vi "ProjectInstance.vi"() -> ()   [LabVIEW 2016, in "test_Setup.lvlib"]
uses:
  test_Setup.lvlib
  <vilib>/addons/_JKI Toolkits/Caraya/classes/Assert/Assert Equal Value_Variant.vi
  <vilib>/addons/_JKI Toolkits/Caraya/classes/Test/Test.lvclass
  <vilib>/addons/_JKI Toolkits/Caraya/classes/Assert/Assert.lvclass
panel:
  out "error out":errorcluster
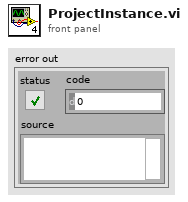
[diagram p1: front panel]
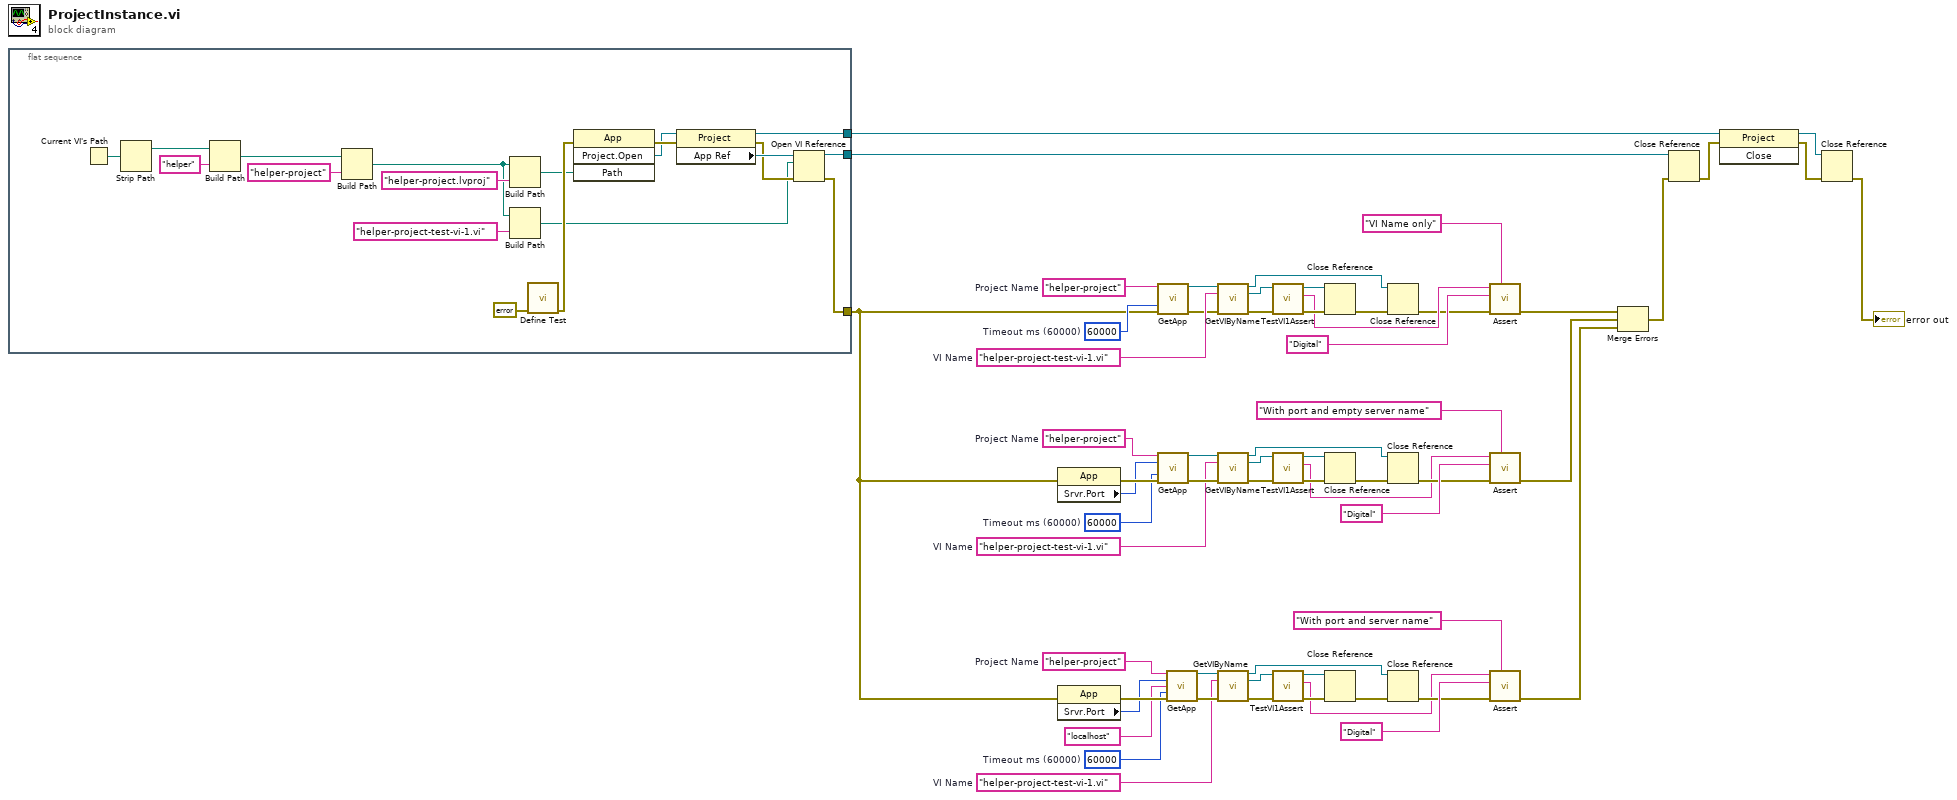
[diagram p0: block diagram]
diagram:
  w1 = "helper-project"  # Project Name
  w2 = "helper-project"  # Project Name
  w3 = "helper-project"  # Project Name
  w7 = 60000  # Timeout ms (60000)
  w10 = "helper-project-test-vi-1.vi"  # VI Name
  w22 = 60000  # Timeout ms (60000)
  w21 = "helper-project-test-vi-1.vi"  # VI Name
  w43 = 60000  # Timeout ms (60000)
  w41 = "helper-project-test-vi-1.vi"  # VI Name
  n1 = flat-sequence {
    tunnel: [w79] -> w5
    tunnel: [w78] -> w61
    tunnel: [w66] -> w60
    frame #0 {
      n2 = Current VI's Path() -> (path=w77:path)
      n3 = Strip Path(path=w77) -> (stripped path=w76:path)  [unwired: 1 out]
      n4 = Build Path(base path=w76, name or relative path="helper") -> (appended path=w74:path)
      n5 = Build Path(base path=w74, name or relative path="helper-project") -> (appended path=w62:path)
      n6 = Build Path(base path=w62, name or relative path="helper-project.lvproj") -> (appended path=w64:path)
      n7 = Build Path(base path=w62, name or relative path="helper-project-test-vi-1.vi") -> (appended path=w63:path)
      n8 = call <vilib>:"Define Test.vi"("error in (no error)"=errorcluster {"status"=FALSE, "code"=0, "source"=""}) -> ("error out"=w69:errorcluster)  [unwired: 10 in]
      n9 = invoke class="App" method="Project.Open"(error in=w69, "Path"=w64) -> (error out=w71:errorcluster, "Project:Open"=w67:refnum<vi>)  [unwired: 2 in, 2 out]
      n10 = property class="Project"(reference=w67, error in=w71) -> (reference out=w66:refnum<vi>, error out=w68:errorcluster, "App Ref"=w70:refnum<vi>)
      n11 = Open VI Reference(application reference (local)=w70, vi path=w63, error in (no error)=w68) -> (vi reference=w78:refnum<vi>, error out=w79:errorcluster)  [unwired: 3 in]
    }
  }
  n12 = property on="Property Node" class="App"(error in=w5) -> (error out=w26:errorcluster, "Srvr.Port"=w23:u32)  [unwired: 1 in, 1 out]
  n13 = property on="Property Node" class="App"(error in=w5) -> (error out=w12:errorcluster, "Srvr.Port"=w9:u32)  [unwired: 1 in, 1 out]
  n14 = call "GetApp.vi"("Project Name (\"\": ThisApplication)"=w3, "Timeout ms (60000)"=w43, "error in (no error)"=w5) -> ("Application Ref"=w40:refnum<vi>, "error out"=w37:errorcluster)  [unwired: 11 in]
  n15 = call "GetApp.vi"("Project Name (\"\": ThisApplication)"=w2, "Port(0:Ignored)"=w23, "Timeout ms (60000)"=w22, "error in (no error)"=w26) -> ("Application Ref"=w30:refnum<vi>, "error out"=w33:errorcluster)  [unwired: 10 in]
  n16 = call "GetApp.vi"("Project Name (\"\": ThisApplication)"=w1, "Port(0:Ignored)"=w9, "Service Name (\"\":localhost)"="localhost" ("Service Name (\"\":localhost)"), "Timeout ms (60000)"=w7, "error in (no error)"=w12) -> ("Application Ref"=w17:refnum<vi>, "error out"=w14:errorcluster)  [unwired: 9 in]
  n17 = call "GetVIByName.vi"("Application Ref in"=w40, "VI Name"=w41, "error in (no error)"=w37) -> ("Application Ref out"=w39:refnum<vi>, "VI Reference"=w38:refnum<vi>, "error out"=w42:errorcluster)  [unwired: 10 in]
  n18 = call "GetVIByName.vi"("Application Ref in"=w30, "VI Name"=w21, "error in (no error)"=w33) -> ("Application Ref out"=w31:refnum<vi>, "VI Reference"=w32:refnum<vi>, "error out"=w29:errorcluster)  [unwired: 10 in]
  n19 = call "GetVIByName.vi"("Application Ref in"=w17, "VI Name"=w10, "error in (no error)"=w14) -> ("Application Ref out"=w16:refnum<vi>, "VI Reference"=w15:refnum<vi>, "error out"=w18:errorcluster)  [unwired: 10 in]
  n20 = call "TestVI1Assert.vi"("error in (no error)"=w42, "VI in"=w38) -> ("error out"=w53:errorcluster, "ClassName"=w51:string, "VI out"=w52:refnum<vi>)  [unwired: 7 in]
  n21 = call "TestVI1Assert.vi"("error in (no error)"=w29, "VI in"=w32) -> ("error out"=w27:errorcluster, "ClassName"=w24:string, "VI out"=w28:refnum<vi>)  [unwired: 7 in]
  n22 = call "TestVI1Assert.vi"("error in (no error)"=w18, "VI in"=w15) -> ("error out"=w20:errorcluster, "ClassName"=w6:string, "VI out"=w19:refnum<vi>)  [unwired: 7 in]
  n23 = Close Reference(reference=w52, error in (no error)=w53) -> (error out=w36:errorcluster)
  n24 = Close Reference(reference=w28, error in (no error)=w27) -> (error out=w34:errorcluster)
  n25 = Close Reference(reference=w19, error in (no error)=w20) -> (error out=w13:errorcluster)
  n26 = Close Reference(reference=w39, error in (no error)=w36) -> (error out=w35:errorcluster)
  n27 = Close Reference(reference=w31, error in (no error)=w34) -> (error out=w25:errorcluster)
  n28 = Close Reference(reference=w16, error in (no error)=w13) -> (error out=w11:errorcluster)
  n29 = call-poly <vilib>:"Assert.vi"("Label"="VI Name only" ("Label (VI Title)"), "error in (no error)"=w35, "Y"="Digital" ("Class Name"), "X"=w51) -> ("error out"=w54:errorcluster)  [unwired: 7 in]
  n30 = call-poly <vilib>:"Assert.vi"("Label"="With port and empty server name" ("Label (VI Title)"), "error in (no error)"=w25, "Y"="Digital" ("Class Name"), "X"=w24) -> ("error out"=w47:errorcluster)  [unwired: 7 in]
  n31 = call-poly <vilib>:"Assert.vi"("Label"="With port and server name" ("Label (VI Title)"), "error in (no error)"=w11, "Y"="Digital" ("Class Name"), "X"=w6) -> ("error out"=w44:errorcluster)  [unwired: 7 in]
  n32 = Merge Errors(w54, w47, w44) -> (w4:errorcluster)
  n33 = Close Reference(reference=w61, error in (no error)=w4) -> (error out=w59:errorcluster)
  n34 = invoke class="Project" method="Close"(reference=w60, error in=w59) -> (reference out=w57:refnum<vi>, error out=w58:errorcluster)  [unwired: 1 in, 1 out]
  n35 = Close Reference(reference=w57, error in (no error)=w58) -> (error out=→"error out":errorcluster)
